vi "Static Write.vi"(8 "error in (no error)":errorcluster, 10 "Waveform":waveform(dbl), 11 "Abs_Waveform in":refnum<class "Abs_Waveform.lvclass">) -> (0 "error out":errorcluster, 3 "Abs_Waveform out":refnum<class "Abs_Waveform.lvclass">)   [LabVIEW 2021, in "Abs_Waveform.lvclass"]
uses:
  Abs_Waveform.lvclass
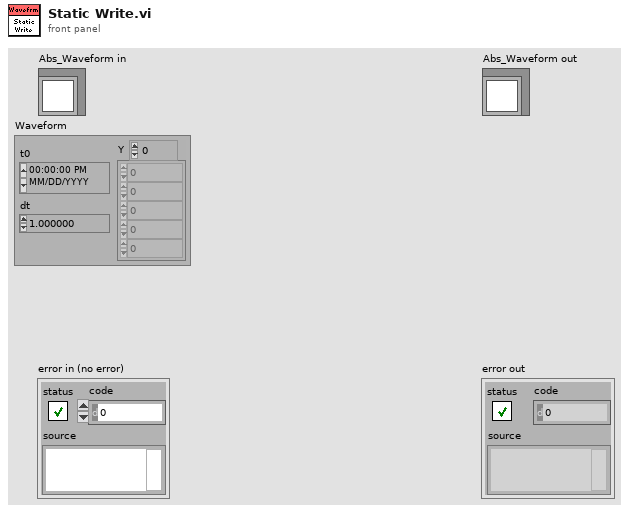
[diagram p1: front panel]
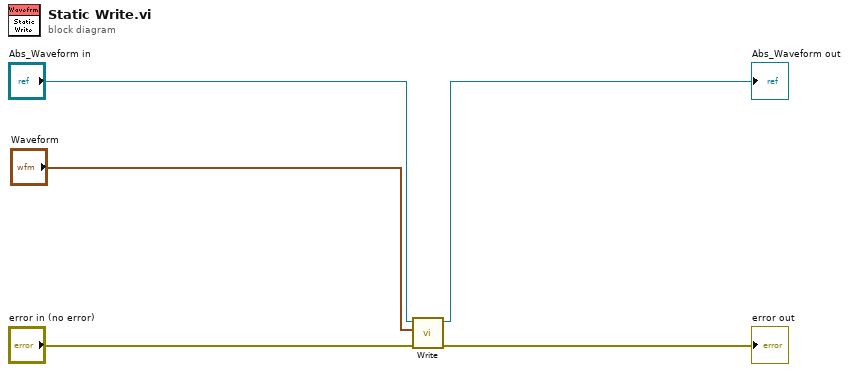
[diagram p0: block diagram]
diagram:
  n1 = call-dynamic "Write.vi"("error in (no error)"="error in (no error)", "Waveform"="Waveform", "Abs_Waveform in"="Abs_Waveform in") -> ("error out"=→"error out":errorcluster, "Abs_Waveform out"=→"Abs_Waveform out":refnum<class "Abs_Waveform.lvclass">)  [unwired: 7 in]
